vi "Get Image Portion.vi"(5 "h":i16, 7 "w":i16, 8 "error in (no error)":errorcluster, 9 "y":i16, 10 "x":i16, 11 "path":path) -> (0 "error out":errorcluster)   [LabVIEW 2020, in "MacroAssert.lvlib"]
uses:
  MacroAssert.lvlib
  System.Drawing
  Win Util/Win Util.lvlib
panel:
  in  "window name":string
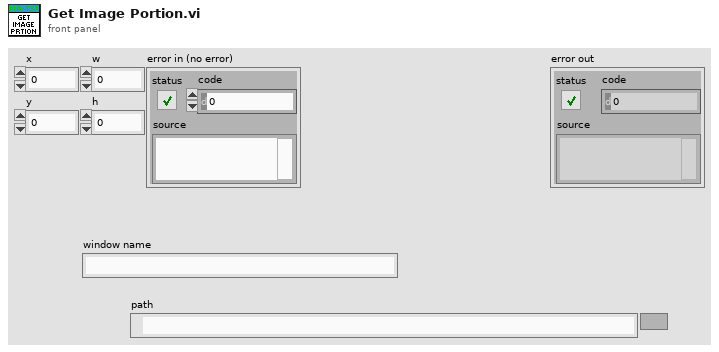
[diagram p1: front panel]
types:
  T1 = typedef "MacroAssert.lvlib/Win Util.lvlib/Window Refnum.ctl" = u64
  T2 = cluster{"left":i16, "top":i16, "right":i16, "bottom":i16}
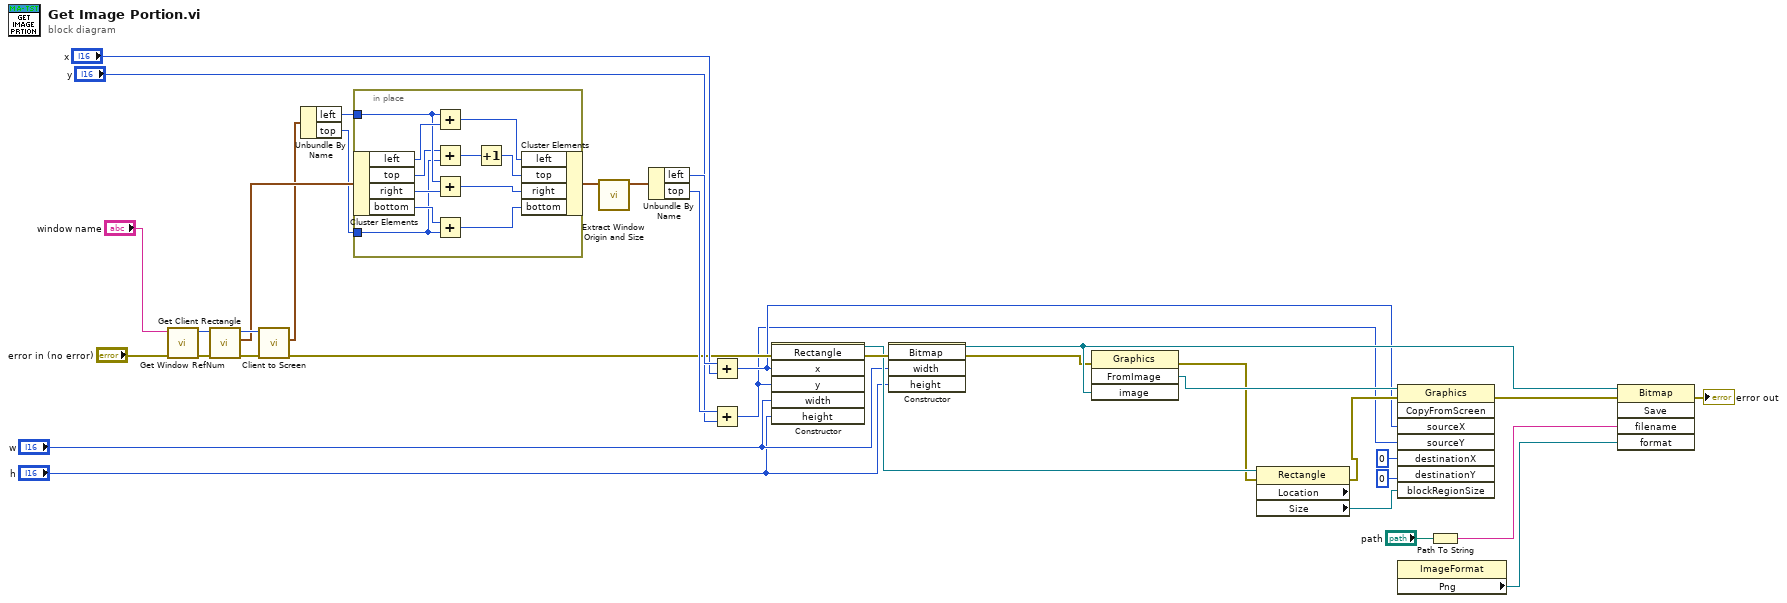
[diagram p0: block diagram]
diagram:
  n1 = call "Get Window RefNum.vi"("error in"="error in (no error)", "window name (\"\")"="window name") -> ("error out"=w36:errorcluster, "window refnum (NaWR)"=w35:T1)  [unwired: 6 in]
  n2 = call "Get Client Rectangle.vi"("error in"=w36, "window refnum (NaWR)"=w35) -> ("error out"=w27:errorcluster, "client rect"=w25:T2, "window refnum out"=w26:T1)  [unwired: 7 in]
  n3 = call "Client to Screen.vi"("error in"=w27, "window refnum (NaWR)"=w26) -> ("error out"=w11:errorcluster, "screen coords"=w1:cluster{"left":i16, "top":i16})  [unwired: 7 in, 1 out]
  n4 = Unbundle By Name(w1) -> ("left"=w24:i16, "top"=w22:i16)
  n5 = in-place {
    in-place-border: w24 -> [w45]
    in-place-border: w22 -> [w42]
    n6 = in-place-cluster #1(w25) -> ("left"=w47:i16, "top"=w44:i16, "right"=w46:i16, "bottom"=w43:i16)
    n7 = Add(x=w45, y=w47) -> (x+y=w41:i16)
    n8 = Add(x=w44, y=w42) -> (x+y=w40:i16)
    n9 = Add(x=w45, y=w46) -> (x+y=w39:i16)
    n10 = Add(x=w43, y=w42) -> (x+y=w38:i16)
    n11 = Increment(x=w40) -> (x+1=w37:i16)
    n12 = in-place-cluster #1("left"=w41, "top"=w37, "right"=w39, "bottom"=w38) -> (w23:T2)
  }
  n13 = call "Extract Window Origin and Size.vi"("window rect"=w23) -> ("window origin"=w28:cluster{"left":i16, "top":i16})  [unwired: 9 in, 1 out]
  n14 = Unbundle By Name(w28) -> ("left"=w32:i16, "top"=w31:i16)
  n15 = Add(x=w32, y="x") -> (x+y=w7:i16)
  n16 = Add(x=w31, y="y") -> (x+y=w6:i16)
  n17 = constructor class="Rectangle"(error in=w11, "x"=w7, "y"=w6, "width"="w", "height"="h") -> (reference out=w33:refnum<k24>, error out=w34:errorcluster)  [unwired: 2 in, 5 out]
  n18 = constructor class="Bitmap"(error in=w34, "width"="w", "height"="h") -> (reference out=w29:refnum<k24>, error out=w10:errorcluster)  [unwired: 2 in, 3 out]
  n19 = invoke class="Graphics" method="FromImage"(error in=w10, "image"=w29) -> (error out=w9:errorcluster, "FromImage"=w14:refnum<k24>)  [unwired: 2 in, 2 out]
  n20 = property class="Rectangle" props=["Location", "Size"](reference=w33, error in=w9) -> (error out=w8:errorcluster, "Size"=w3:refnum<k24>)  [unwired: 2 out]
  n21 = invoke class="Graphics" method="CopyFromScreen"(reference=w14, error in=w8, "sourceX"=w7, "sourceY"=w6, "destinationX"=0, "destinationY"=0, "blockRegionSize"=w3) -> (error out=w16:errorcluster)  [unwired: 1 in, 7 out]
  n22 = property class="ImageFormat"() -> ("Png"=w17:refnum<k24>)  [unwired: 2 in, 2 out]
  n23 = Path To String(path="path") -> (string=w30:string)
  n24 = invoke class="Bitmap" method="Save"(reference=w29, error in=w16, "filename"=w30, "format"=w17) -> (error out=→"error out":errorcluster)  [unwired: 1 in, 4 out]
